vi "电导率电极校准.vi"() -> ()   [LabVIEW 2016, in "国弘多参数.lvlib"]
panel:
  out "提示":string
  in  "第二点通过校正":bool
  in  "第一点通过校正":bool
  in  "第二点校正":bool
  in  "第一点校正":bool
  out "标液2":dbl
  out "标液1":dbl
  out "当前读取值":dbl
  out "偏移值补偿":dbl
  out "电极系数":dbl
  out "温度补偿系数":dbl caption="温度系数"
  # "电导率电极设定"
  # "uS/cm"
  # "%"
  # "-1"
  # "uS/cm"
  # "cm"
  # "电极校正"
  # "标准液值:"
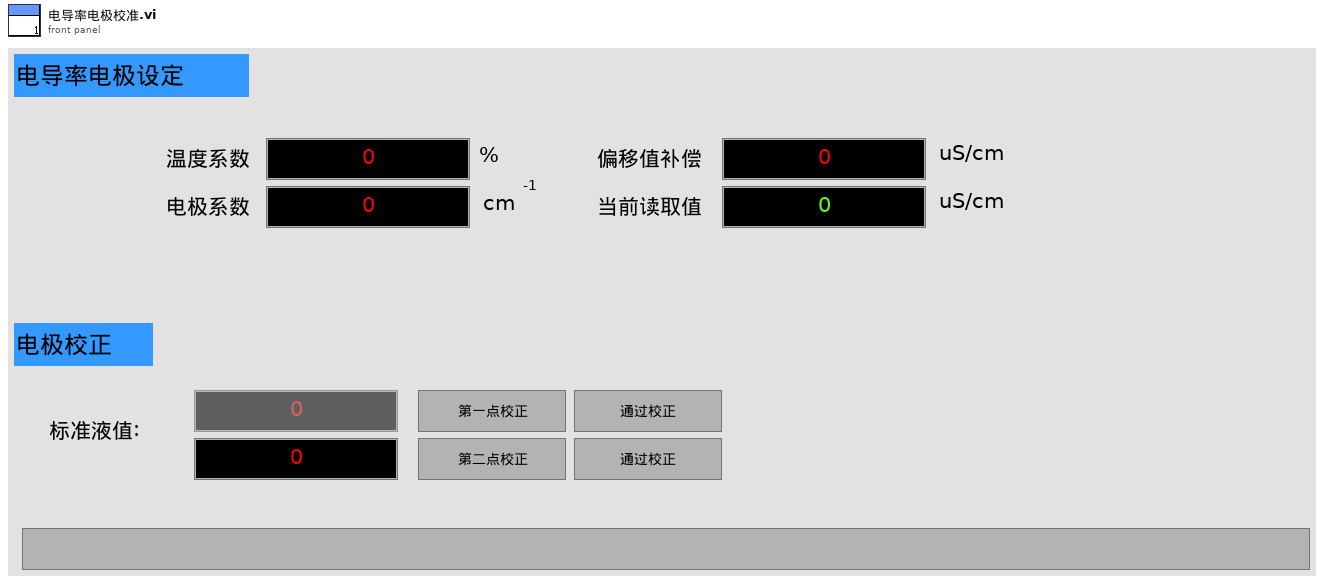
[diagram p1: front panel]
types:
  T1 = cluster{"电极状态标志":u16, "电极型号标志":u16, "电导率测量值":sgl, "温度测量值":sgl, "电导率信号值":sgl, "温度信号值":sgl, "温度补偿系数":sgl, "电导率偏移修正值":sgl, "温度偏移修正值":sgl, "手动温度补偿值":sgl, "电导率电极零点":sgl, "电导率电极斜率":sgl, "命令滤波设定":u16, "温度模式":enum16{"ATC", "MTC"}, "生产批次":u16, "电极序号":u16, "串口地址":u16, "串口波特率":enum16{"9600", "19200", "115200"}, "串口校验位":enum16{"NONE", "ODD", "EVEN"}, "串口停止位":enum16{"1bit", "2bit"}, "第一点标准值":sgl, "第二点标准值":sgl}
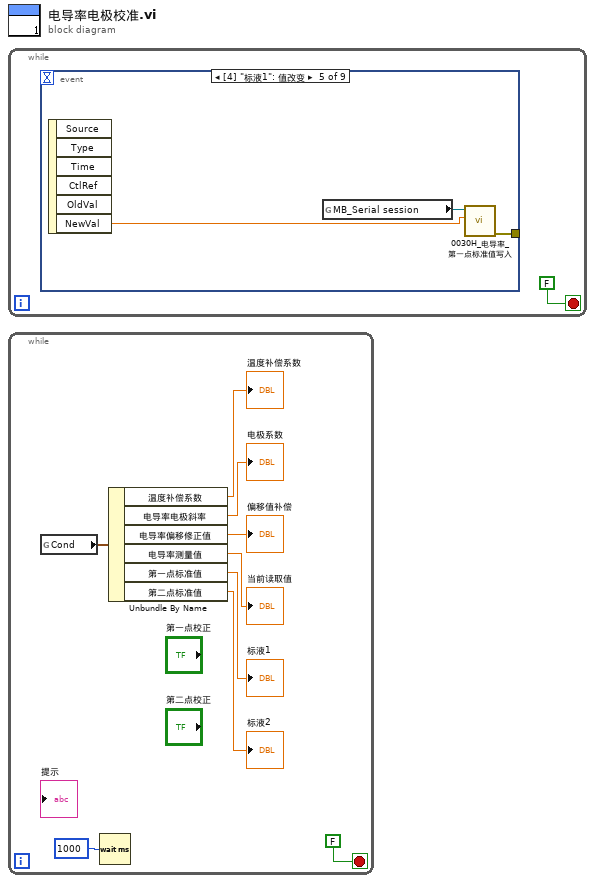
[diagram p0: block diagram]
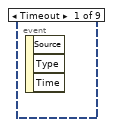
[diagram p2: hidden frame]
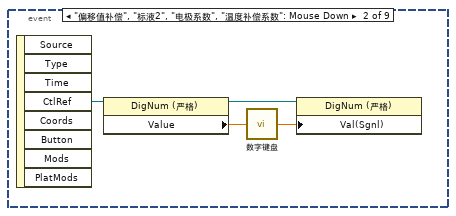
[diagram p3: hidden frame]
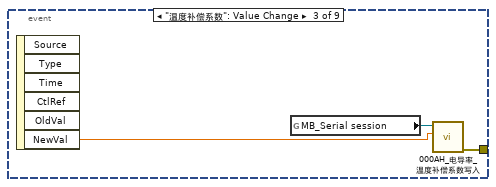
[diagram p4: hidden frame]
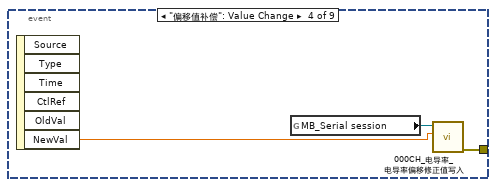
[diagram p5: hidden frame]
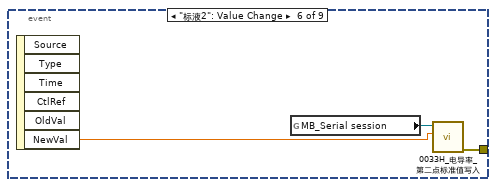
[diagram p6: hidden frame]
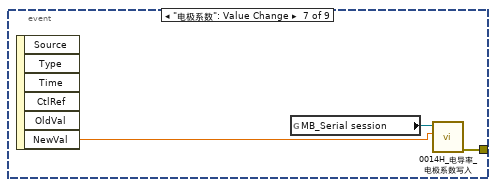
[diagram p7: hidden frame]
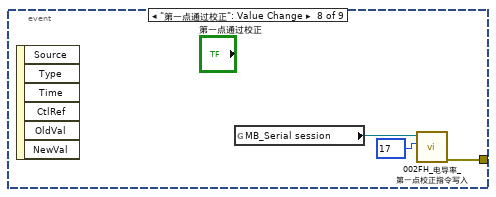
[diagram p8: hidden frame]
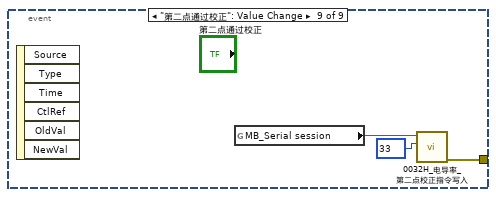
[diagram p9: hidden frame]
diagram:
  n1 = while {
    stop <- FALSE stop-if-true
    n2 = event shown="[4] \"标液1\": 值改变" {
      selector: _ -> [_ _ _ _ _ _ _ _ _]
      dyn-events: _ -> [_ _ _ _ _ _ _ _ _]
      timeout: _ -> [_ _ _ _ _ _ _ _ _]
      tunnel: [_ _ w6 w9 w12 w17 w20 w23 w26] -> _
      event Timeout {
        n3 = event-data() -> ()  [unwired: 1 in, 3 out]
      }
      event "偏移值补偿", "标液2", "电极系数", "温度补偿系数": Mouse Down {
        n4 = event-data() -> ("CtlRef"=w2:refnum<vi>)  [unwired: 1 in, 7 out]
        n5 = property class="DigNum (严格)"(reference=w2) -> (reference out=w3:refnum<vi>, "Value"=w4:dbl)  [unwired: 1 in, 1 out]
        n6 = call "数字键盘.vi"("OldNumber"=w4) -> ("NewNumber"=w5:sgl)
        n7 = property class="DigNum (严格)"(reference=w3, "Val(Sgnl)"=w5) -> ()  [unwired: 1 in, 2 out]
      }
      event "温度补偿系数": Value Change {
        n8 = event-data() -> ("NewVal"=w7:dbl)  [unwired: 1 in, 5 out]
        n9 = global read "过程全局变量.vi" "MB_Serial session"() -> (w8:refnum<class "MB_Master_Serial.lvclass">)
        n10 = call "000AH_电导率_温度补偿系数写入.vi"("数值"=w7, "MB_Serial session in"=w8) -> ("error out"=w6:errorcluster)  [unwired: 8 in, 1 out]
      }
      event "偏移值补偿": Value Change {
        n11 = event-data() -> ("NewVal"=w10:dbl)  [unwired: 1 in, 5 out]
        n12 = global read "过程全局变量.vi" "MB_Serial session"() -> (w11:refnum<class "MB_Master_Serial.lvclass">)
        n13 = call "000CH_电导率_电导率偏移修正值写入.vi"("数值"=w10, "MB_Serial session in"=w11) -> ("error out"=w9:errorcluster)  [unwired: 8 in, 1 out]
      }
      event "标液1": Value Change {
        n14 = event-data() -> ("NewVal"=w13:dbl)  [unwired: 1 in, 5 out]
        n15 = global read "过程全局变量.vi" "MB_Serial session"() -> (w14:refnum<class "MB_Master_Serial.lvclass">)
        n16 = call "0030H_电导率_第一点标准值写入.vi"("数值"=w13, "MB_Serial session in"=w14) -> ("error out"=w12:errorcluster)  [unwired: 8 in, 1 out]
      }
      event "标液2": Value Change {
        n17 = event-data() -> ("NewVal"=w15:dbl)  [unwired: 1 in, 5 out]
        n18 = global read "过程全局变量.vi" "MB_Serial session"() -> (w16:refnum<class "MB_Master_Serial.lvclass">)
        n19 = call "0033H_电导率_第二点标准值写入.vi"("数值"=w15, "MB_Serial session in"=w16) -> ("error out"=w17:errorcluster)  [unwired: 8 in, 1 out]
      }
      event "电极系数": Value Change {
        n20 = event-data() -> ("NewVal"=w18:dbl)  [unwired: 1 in, 5 out]
        n21 = global read "过程全局变量.vi" "MB_Serial session"() -> (w19:refnum<class "MB_Master_Serial.lvclass">)
        n22 = call "0014H_电导率_电极系数写入.vi"("数值"=w18, "MB_Serial session in"=w19) -> ("error out"=w20:errorcluster)  [unwired: 8 in, 1 out]
      }
      event "第一点通过校正": Value Change {
        n23 = event-data() -> ()  [unwired: 1 in, 6 out]
        n24 = global read "过程全局变量.vi" "MB_Serial session"() -> (w22:refnum<class "MB_Master_Serial.lvclass">)
        n25 = call "002FH_电导率_第一点校正指令写入.vi"("数值"=u16 17, "MB_Serial session in"=w22) -> ("error out"=w23:errorcluster)  [unwired: 8 in, 1 out]
      }
      event "第二点通过校正": Value Change {
        n26 = event-data() -> ()  [unwired: 1 in, 6 out]
        n27 = global read "过程全局变量.vi" "MB_Serial session"() -> (w24:refnum<class "MB_Master_Serial.lvclass">)
        n28 = call "0032H_电导率_第二点校正指令写入.vi"("数值"=u16 33, "MB_Serial session in"=w24) -> ("error out"=w26:errorcluster)  [unwired: 8 in, 1 out]
      }
    }
  }
  n29 = while {
    stop <- FALSE stop-if-true
    n30 = global read "过程全局变量.vi" "Cond"() -> (w33:T1)
    n31 = Wait (ms)(milliseconds to wait=u32 1000 ("等待时间（毫秒）")) -> ()  [unwired: 1 out]
    n32 = Unbundle By Name(w33) -> ("温度补偿系数"=→"温度补偿系数":sgl, "电导率电极斜率"=→"电极系数":sgl, "电导率偏移修正值"=→"偏移值补偿":sgl, "电导率测量值"=→"当前读取值":sgl, "第一点标准值"=→"标液1":sgl, "第二点标准值"=→"标液2":sgl)
  }
